vi "Get Assembly Version.vi"(8 "error in (no error)":errorcluster, 11 "Parse Presentation in":refnum<class "Parse Presentation.lvclass">) -> (0 "error out":errorcluster, 3 "Parse Presentation out":refnum<class "Parse Presentation.lvclass">)   [LabVIEW 2015, in "Parse Presentation.lvclass"]
uses:
  Parse Presentation.lvclass
  D:/Metis Automation/ppt-parsing/LabVIEW/DLL/ParsePpt.dll
  DLL/ParsePpt.dll
  Parse Presentation.lvclass/Parse Presentation.ctl
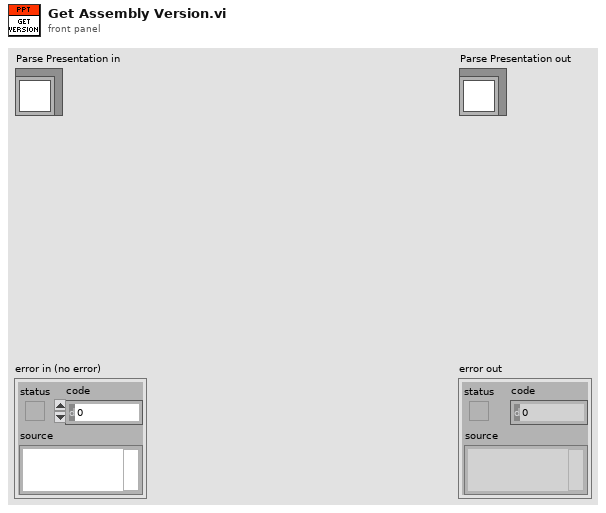
[diagram p1: front panel]
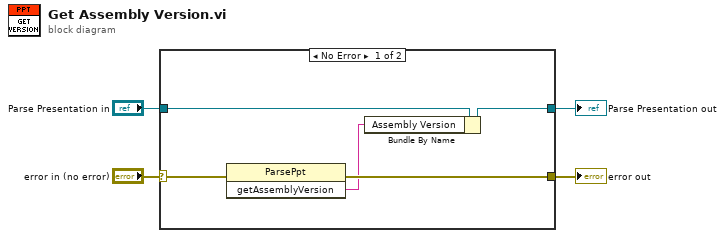
[diagram p0: block diagram]
diagram:
  n1 = case shown="No Error" "error in (no error)" {
    selector: "error in (no error)" -> [w8 w11]
    tunnel: [w7 w11] -> w3
    tunnel: [w6 w10] -> w1
    tunnel: "Parse Presentation in" -> [w9 w10]
    frame No Error {
      n2 = invoke class="ParsePpt" method="getAssemblyVersion"(error in=w8) -> (error out=w7:errorcluster, "getAssemblyVersion"=w5:string)  [unwired: 2 in, 1 out]
      n3 = Bundle By Name(cluster=w9, "Assembly Version"=w5) -> (w6:refnum<class "Parse Presentation.lvclass">)
    }
    frame Error {
    }
  }
  "error out" <- w3
  "Parse Presentation out" <- w1
